vi "Deney 2.vi"() -> ()   [LabVIEW 2018]
panel:
  out "While Counter":i32
  in  "CHART MODE":T1(ring)
  in  "?":bool
  out "Waveform Chart":dbl(graph)
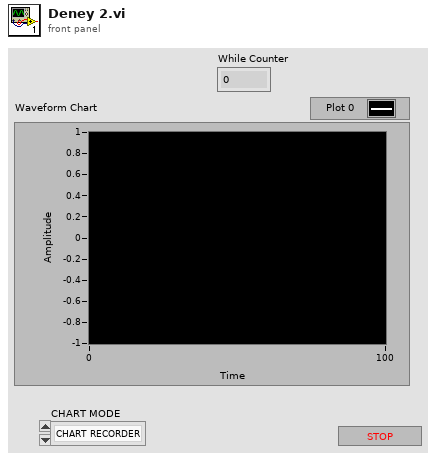
[diagram p1: front panel]
types:
  T1 = enum16{"CHART RECORDER", "OSCILLOSCOPE", "SWEEP"}
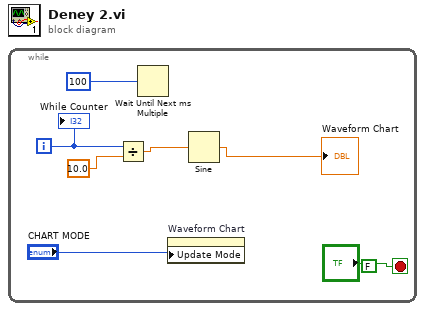
[diagram p0: block diagram]
diagram:
  n1 = while {
    i -> [w3]
    stop <- "?" stop-if-true
    (unwired) FALSE
    n2 = Divide(x=w3, y=10.0) -> (x/y=w2:dbl)
    n3 = Wait Until Next ms Multiple(millisecond multiple=100) -> ()  [unwired: 1 out]
    n4 = property on="Waveform Chart" class="WFChart (strict)"("Update Mode"="CHART MODE") -> ()  [unwired: 2 in, 2 out]
    n5 = Sine(x=w2) -> (sin(x)=→"Waveform Chart":dbl)
    "While Counter" <- w3
  }
